vi "queuesWithNavX.vi"() -> ()   [LabVIEW 2017]
uses:
  <vilib>/myRIO/Common/Instrument Driver Framework/Utilities/typedefs/FPGA Ref Manager Action Enum.ctl
  <vilib>/myRIO/Instrument Drivers/Onboard IO/I2C/typedefs/I2C Reference.ctl
  <vilib>/myRIO/Common/Instrument Driver Framework/Utilities/typedefs/myRIO Generic Hardware Reference.ctl
  <vilib>/myRIO/Common/Instrument Driver Framework/Utilities/typedefs/Hardware Version Enum.ctl
  <vilib>/myRIO/Common/Instrument Driver Framework/Utilities/typedefs/myRIO v1.0 Reference.ctl
  <vilib>/myRIO/Common/Instrument Driver Framework/Utilities/typedefs/Generic FPGA Reference.ctl
  <vilib>/myRIO/Common/Instrument Driver Framework/myRIO v1.0/I2C/typedefs/I2C Channels Enum.ctl
  <vilib>/myRIO/Instrument Drivers/Onboard IO/I2C/typedefs/I2C Configuration.ctl
  <vilib>/myRIO/Instrument Drivers/Onboard IO/I2C/typedefs/I2C Transfer Rate.ctl
  <vilib>/userdefined/High Color/nirio_resource_hc.ctl
  <vilib>/myRIO/Common/Instrument Driver Framework/myRIO v1.0/I2C/vis/myRIO v1.1 Open I2C.vi
  <vilib>/myRIO/Common/Instrument Driver Framework/Utilities/vis/Validate Channels.vi
  <vilib>/myRIO/Common/Instrument Driver Framework/myRIO v1.0/I2C/vis/myRIO v1.0 Reserve I2C.vi
  <vilib>/myRIO/Common/Instrument Driver Framework/myRIO v1.0/I2C/vis/myRIO v1.0 Close I2C.vi
  <vilib>/myRIO/Common/Instrument Driver Framework/myRIO v1.0/I2C/vis/myRIO v1.0 Build MUX Configuration I2C.vi
  <vilib>/myRIO/Common/Instrument Driver Framework/myRIO v1.0/Resource Manager/vis/myRIO v1.0 Reserve Channel List.vi
  <vilib>/myRIO/Common/Instrument Driver Framework/myRIO v1.0/I2C/vis/myRIO v1.0 Unreserve I2C.vi
  <vilib>/myRIO/Common/Instrument Driver Framework/myRIO v1.0/Resource Manager/vis/myRIO v1.0 Create Configuration List.vi
  <vilib>/myRIO/Common/Instrument Driver Framework/myRIO v1.0/Resource Manager/vis/myRIO v1.0 Reserve Channel.vi
  <vilib>/myRIO/Common/Instrument Driver Framework/myRIO v1.0/Resource Manager/vis/myRIO v1.0 Unreserve Channel.vi
  <vilib>/myRIO/Common/Instrument Driver Framework/myRIO v1.0/Resource Manager/vis/myRIO v1.0 Unreserve Channel List.vi
  <vilib>/myRIO/Common/Instrument Driver Framework/myRIO v1.0/Resource Manager/vis/myRIO v1.0 Build Mutex Name.vi
  <vilib>/Utility/VariantDataType/GetNumericInfo.vi
  <vilib>/Utility/error.llb/Error Cluster From Error Code.vi
  <vilib>/myRIO/Common/Instrument Driver Framework/myRIO v1.0/myRIO v1.1 Open.vi
  <vilib>/myRIO/Common/Instrument Driver Framework/Utilities/vis/IO Manager.vi
  <vilib>/myRIO/Common/Instrument Driver Framework/Utilities/vis/Configuration Manager.vi
  <vilib>/myRIO/Common/Instrument Driver Framework/myRIO v1.0/Resource Manager/vis/myRIO v1.0 Configure IO.vi
  <vilib>/myRIO/Common/Instrument Driver Framework/myRIO v1.0/myRIO v1.0 Close.vi
  <vilib>/myRIO/Common/Instrument Driver Framework/myRIO v1.0/I2C/vis/myRIO v1.0 Shutdown I2C.vi
  <vilib>/myRIO/Instrument Drivers/Onboard IO/I2C/vis/myRIO I2C Open.xnode
  <vilib>/myRIO/Instrument Drivers/Onboard IO/I2C/I2C.lvlib
panel:
  out "value Z 2":ext
  out "value Z":ext
  out "main":ext
  out "right":dbl
  out "left":dbl
  in  "angle":ext format="%#_13g"
  out "zero angle":ext
  out "error out":errorcluster
  in  "error in (no error)":errorcluster
  in  "Stop Button":bool
  out "axis Z":ext
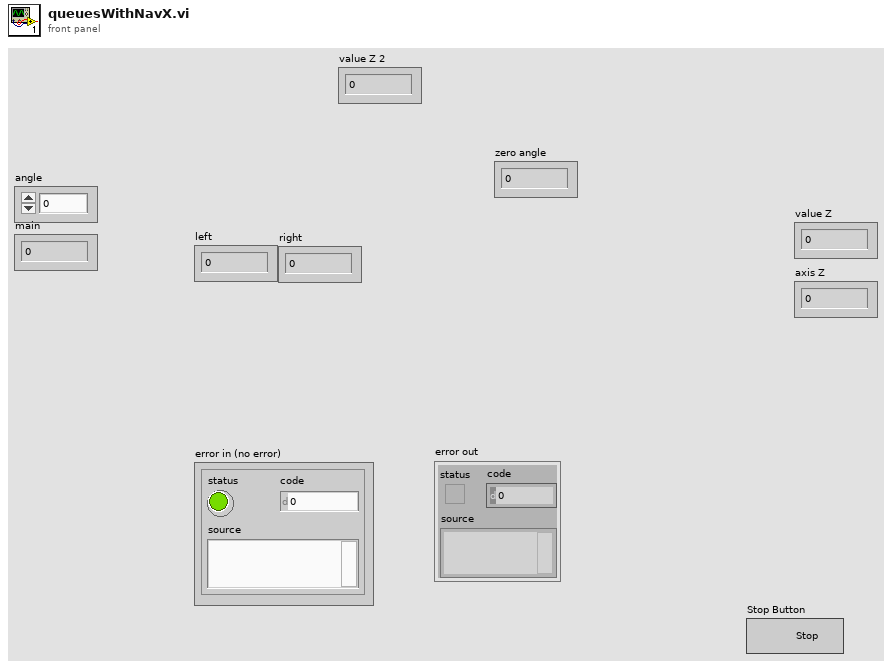
[diagram p1: front panel]
types:
  T1 = typedef "FPGA Ref Manager Action Enum.ctl" = enum16{"Get", "Set", "Reset"}
  T2 = typedef "I2C.lvlib/I2C Reference.ctl" = cluster{"myRIO Reference":T3, "I2C Channels Enum":T7, "I2C Configuration":T8}
  T3 = typedef "myRIO Generic Hardware Reference.ctl" = cluster{"myRIO Model":T4, "myRIO Hardware Reference":T5}
  T4 = typedef "Hardware Version Enum.ctl" = enum16{"Unknown", "myRIO-1900", "myRIO-1950", "roboRIO", "NI ELVIS RIO CM"}
  T5 = typedef "myRIO v1.0 Reference.ctl" = cluster{"Generic FPGA Reference":T6, "Allow multiple opens":bool}
  T6 = typedef "Generic FPGA Reference.ctl" = refnum<k20>
  T7 = typedef "I2C Channels Enum.ctl" = enum16{"Not Connected", "A/I2C", "B/I2C", "I2C/I2C"}
  T8 = typedef "I2C.lvlib/I2C Configuration.ctl" = cluster{"I2C Transfer Rate":T9}
  T9 = typedef "I2C.lvlib/I2C Transfer Rate.ctl" = enum16{"Standard mode (100 kbps)", "Fast mode (400 kbps)"}
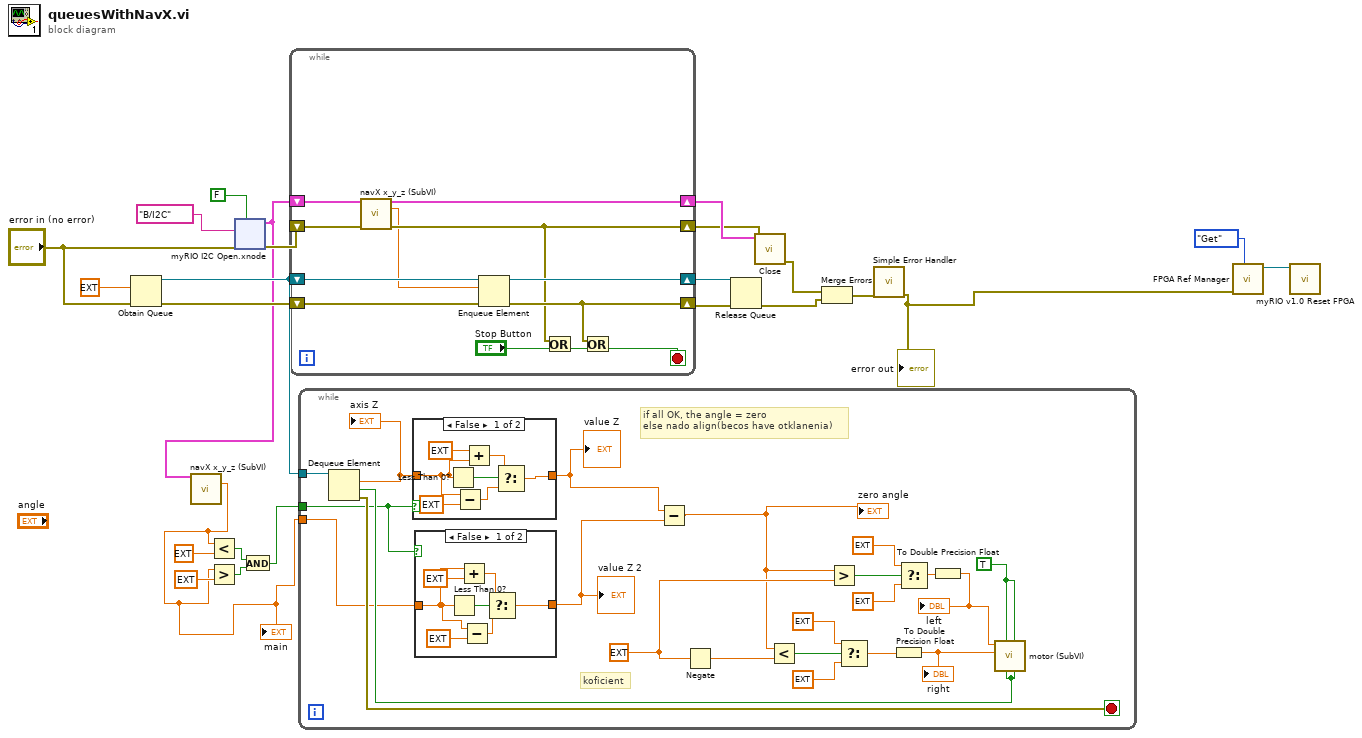
[diagram p0: block diagram]
diagram:
  n1 = Obtain Queue(element data type=ext 0.0 ("value Z"), error in (no error)="error in (no error)") -> (queue out=w11:refnum<queue>, error out=w24:errorcluster)  [unwired: 3 in, 1 out]
  n2 = xnode "myRIO I2C Open.xnode"("error in (no error)"="error in (no error)", "Allow multiple opens?"=FALSE, "Channel Name"=tag "B/I2C") -> ("error out"=w17:errorcluster, "I2C Ref Out"=w7:T2)
  n3 = call "navX x_y_z (SubVI).vi"("I2C Ref Out in"=w7) -> ("value Z"=w4:ext)  [unwired: 10 in, 4 out]
  "main" <- w4
  n4 = Less?(x=w4, y=ext 90.0) -> (x < y?=w2:bool)
  n5 = Greater?(x=w4, y=ext -90.0) -> (0:w5:bool)
  n6 = And(x=w2, y=w5) -> (x .and. y?=w1:bool)
  n7 = while {
    shift-right: [w29] -> w22
    shift-left: w24 -> [w35]
    shift-right: [w34] -> w23
    shift-left: w11 -> [w36]
    shift-right: [w31] -> w18
    shift-left: w7 -> [w32]
    shift-right: [w26] -> w16
    shift-left: w17 -> [w27]
    stop <- w30 stop-if-true
    n8 = call "navX x_y_z (SubVI).vi"("I2C Ref Out in"=w32, "error in (no error)"=w27) -> ("I2C Ref Out out"=w31:T2, "value Z"=w25:ext, "error out"=w26:errorcluster)  [unwired: 9 in, 2 out]
    n9 = Enqueue Element(queue=w36, element=w25, error in (no error)=w35) -> (queue out=w34:refnum<queue>, error out=w29:errorcluster)  [unwired: 1 in, 1 out]
    n10 = Or(x=w26, y="Stop Button") -> (x .or. y?=w28:bool)
    n11 = Or(x=w29, y=w28) -> (x .or. y?=w30:bool)
  }
  n12 = while {
    tunnel: w11 -> [w58]
    tunnel: w4 -> [w40]
    tunnel: w1 -> [w39]
    stop <- w57 stop-if-true
    w46 = TRUE ("M0 (Pin 21)")
    w50 = ext 1.0 ("y")
    # "koficient"
    # "if all OK, the angle = zero\nelse nado align(becos have otklanenia)"
    n13 = Dequeue Element(queue=w58) -> (element=w42:ext, timed out?=w45:bool, error out=w57:errorcluster)  [unwired: 2 in, 1 out]
    "axis Z" <- w42
    n14 = case shown="False" w39 {
      tunnel: [w72 w74] -> w43
      tunnel: w42 -> [w68 w74]
      frame False {
        n15 = Less Than 0?(x=w68) -> (x < 0?=w73:bool)
        n16 = Subtract(x=w68, y=ext 180.0) -> (x-y=w69:ext)
        n17 = Add(x=ext 180.0, y=w68) -> (x+y=w71:ext)
        n18 = Select(t=w71, s=w73, f=w69) -> (s? t:f=w72:ext)
      }
      frame True {
      }
    }
    "value Z" <- w43
    n19 = case shown="False" w39 {
      tunnel: [w64 w66] -> w41
      tunnel: w40 -> [w61 w66]
      frame False {
        n20 = Less Than 0?(x=w61) -> (x < 0?=w65:bool)
        n21 = Add(x=w61, y=ext 180.0) -> (x+y=w63:ext)
        n22 = Subtract(x=w61, y=ext 180.0) -> (x-y=w62:ext)
        n23 = Select(t=w63, s=w65, f=w62) -> (s? t:f=w64:ext)
      }
      frame True {
      }
    }
    "value Z 2" <- w41
    n24 = Subtract(x=w43, y=w41) -> (x-y=w44:ext)
    "zero angle" <- w44
    n25 = Negate(x=w50) -> (-x=w49:ext)
    n26 = Less?(x=w44, y=w49) -> (x < y?=w53:bool)
    n27 = Greater?(x=w44, y=w50) -> (0:w56:bool)
    n28 = Select(t=ext 0.2 ("y"), s=w53, f=ext 0.4 ("y")) -> (s? t:f=w47:ext)
    n29 = To Double Precision Float(number=w47) -> (double precision float=w38:dbl)
    "right" <- w38
    n30 = Select(t=ext 0.2 ("y"), s=w56, f=ext 0.4 ("y")) -> (s? t:f=w48:ext)
    n31 = To Double Precision Float(number=w48) -> (double precision float=w37:dbl)
    "left" <- w37
    n32 = call "motor (SubVI).vi"("M1 (Pin 26)"=w45, "M1 (Pin 25)"=w46, "M0 (Pin 23)"=w45, "M0 (Pin 21)"=w46, "PWM1"=w38, "PWM0"=w37) -> ()  [unwired: 5 in, 1 out]
  }
  n33 = Release Queue(queue=w23, error in (no error)=w22) -> (error out=w13:errorcluster)  [unwired: 1 in, 2 out]
  n34 = call <vilib>:"Close.vi"("error in (no error)"=w16, "I2C Ref In"=w18) -> ("error out"=w14:errorcluster)  [unwired: 9 in]
  n35 = Merge Errors(w14, w13) -> (w15:errorcluster)
  n36 = call <vilib>:"Simple Error Handler.vi"("error in (no error)"=w15) -> ("error out"=w8:errorcluster)  [unwired: 4 in, 4 out]
  "error out" <- w8
  n37 = call <vilib>:"FPGA Ref Manager.vi"("Action"=FPGA_Ref_Manager_Action_Enum."Get" ("Ref Counter Action Enum"), "error in (no error)"=w8) -> ("Generic FPGA Reference out"=w10:T6)  [unwired: 7 in, 1 out]
  n38 = call <vilib>:"myRIO v1.0 Reset FPGA.vi"("Generic FPGA Reference in"=w10) -> ()  [unwired: 9 in, 2 out]
